vi "Read U64.vi"(11 "Event in":refnum<class "Event U64.lvclass">) -> (2 "U64":u64, 3 "Event out":refnum<class "Event U64.lvclass">)   [LabVIEW 2016, in "Event Source.lvlib" / "Event U64.lvclass"]
uses:
  Event U64.lvclass
  Event U64.lvclass/Event U64.ctl
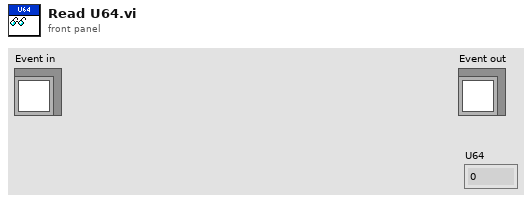
[diagram p1: front panel]
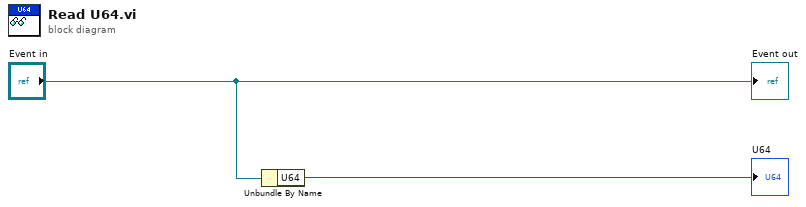
[diagram p0: block diagram]
diagram:
  n1 = Unbundle By Name("Event in") -> ("U64"=→"U64":u64)
  "Event out" <- "Event in"
